vi "onAssertionSlippage.vi"(7 "Peel":refnum<class "GUID.lvclass">, 10 "Properties.Assert":refnum<class "Properties.Assert.lvclass">) -> (0 "error out":errorcluster, 2 "Properties.Assert out":refnum<class "Properties.Assert.lvclass">)   [LabVIEW 2021, in "Bananas.lvlib" / "GUID.lvclass"]
uses:
  GUID.lvclass
  <vilib>/addons/_JKI Toolkits/Caraya/classes/Properties.Assert/Properties.Assert.lvclass
  C:/Program Files (x86)/National Instruments/LabVIEW 2021/vi.lib/addons/_JKI Toolkits/Caraya/classes/Properties/Properties.lvclass
  GUID.lvclass/GUID.ctl
  <vilib>/addons/_JKI Toolkits/Caraya/classes/Properties/Properties.lvclass
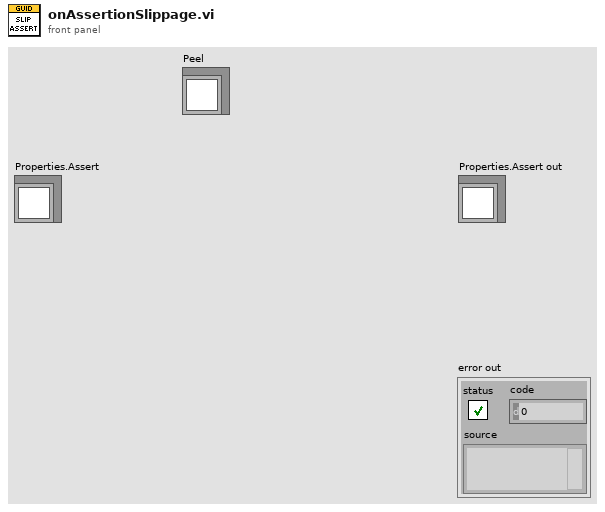
[diagram p1: front panel]
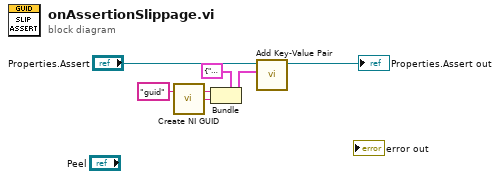
[diagram p0: block diagram]
diagram:
  n1 = call <vilib>:"Create NI GUID.vi"() -> ("NI GUID"=w3:string)
  n2 = Bundle(cluster=cluster{"key":string, "value":variant} {"key"="", "value"=variant} ("entry"), "key"="guid", "value"=w3) -> (w5:cluster{"key":string, "value":variant})
  n3 = call <vilib>:"Add Key-Value Pair.vi"("entry"=w5, "Properties in"="Properties.Assert") -> ("Properties out"=→"Properties.Assert out":refnum<class "Properties.Assert.lvclass">)  [unwired: 8 in, 1 out]
